vi "Write Index.vi"(10 "Index":i32, 11 "(Index_Pointer) In":refnum<class "Index_Pointer.lvclass">) -> (3 "(Index_Pointer) Out":refnum<class "Index_Pointer.lvclass">)   [LabVIEW 2020, in "Index_Pointer.lvclass"]
uses:
  Index_Pointer.lvclass
  Index_Pointer.lvclass/Index_Pointer.ctl
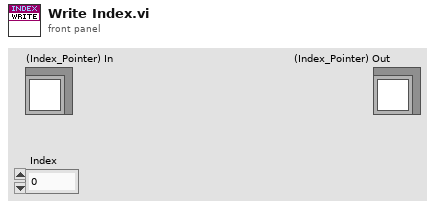
[diagram p1: front panel]
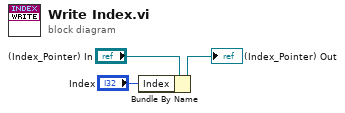
[diagram p0: block diagram]
diagram:
  n1 = Bundle By Name(cluster="(Index_Pointer) In", "Index"="Index") -> (→"(Index_Pointer) Out":refnum<class "Index_Pointer.lvclass">)
